vi "high_field_probe_choose_peaks.vi"() -> ()   [LabVIEW 2011]
uses:
  <vilib>/express/express arith-compare/Formula/XNode/ExpressFormulaBlockNode.xnode
  <vilib>/Analysis/NI_AALBase.lvlib
panel:
  out "Zero Ratio":dbl
  out "normalized amplitude":dbl
  out "average power":dbl
  in  "Shutter":bool
  out "Time":string
  in  "3 peak":dbl[](array[numeric])=[0.02, 0.3, 0.12, 0.005, 0.9, 0.012, 0.03, 1.4, 0.12, 0.0]
  in  "3 peaks?":bool
  out "Waveform Chart 2":dbl(graph)
  out "best fit":dbl[](array[numeric])
  in  "Set Zero Peaks":bool
  out "Peak 2 Amp":dbl
  out "Peak 1 Amp":dbl
  out "Polarization":dbl
  out "Peak Ratio":dbl
  out "XY Graph":cluster{dbl[], dbl[]}[](graph)
  in  "Peak 2 at Zero":dbl=1.0
  in  "Peak 1 at Zero":dbl=1.0
  in  "2 peak":dbl[](array[numeric])=[0.02, 0.3, 0.12, 0.03, 1.4, 0.12, 0.0, 1.4, 0.12]
  in  "stop":bool
  in  "Center Freq":dbl=1000.0
  in  "Voltage Sweep Range":dbl=2.2
  out "Set Voltage":dbl
  in  "threshold":dbl=0.0005
  in  "rate":dbl=20000.0
  in  "number of samples":i32=500
  out "data":dynamicdata(graph)
  out "Waveform Chart":dbl(graph)
  out "amplitude":dbl
  out "frequency":dbl
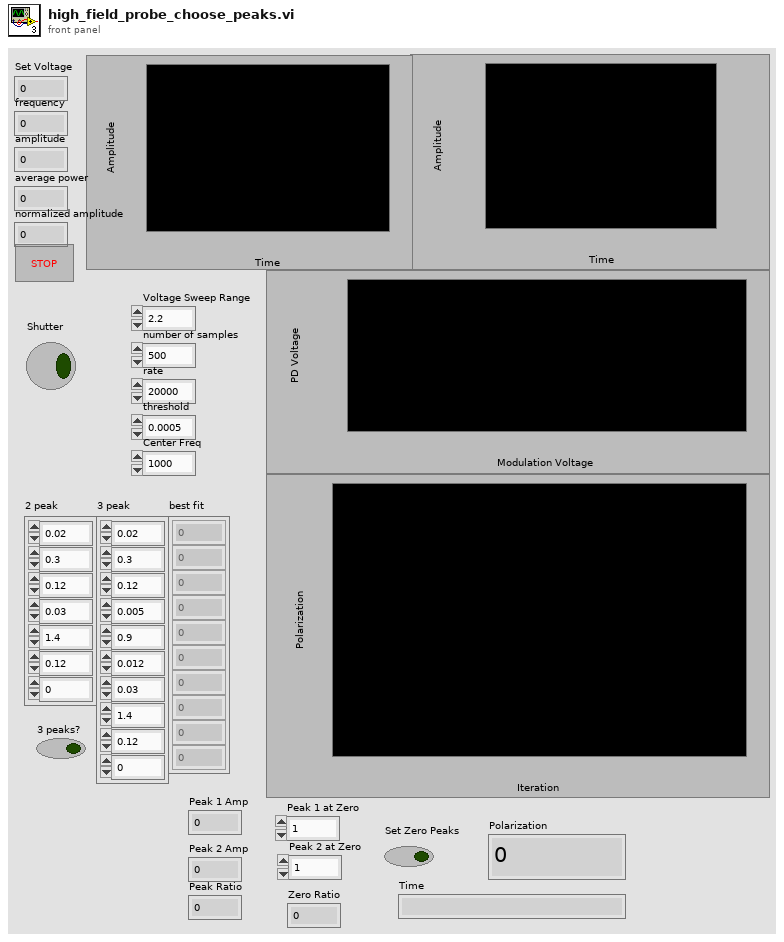
[diagram p1: front panel]
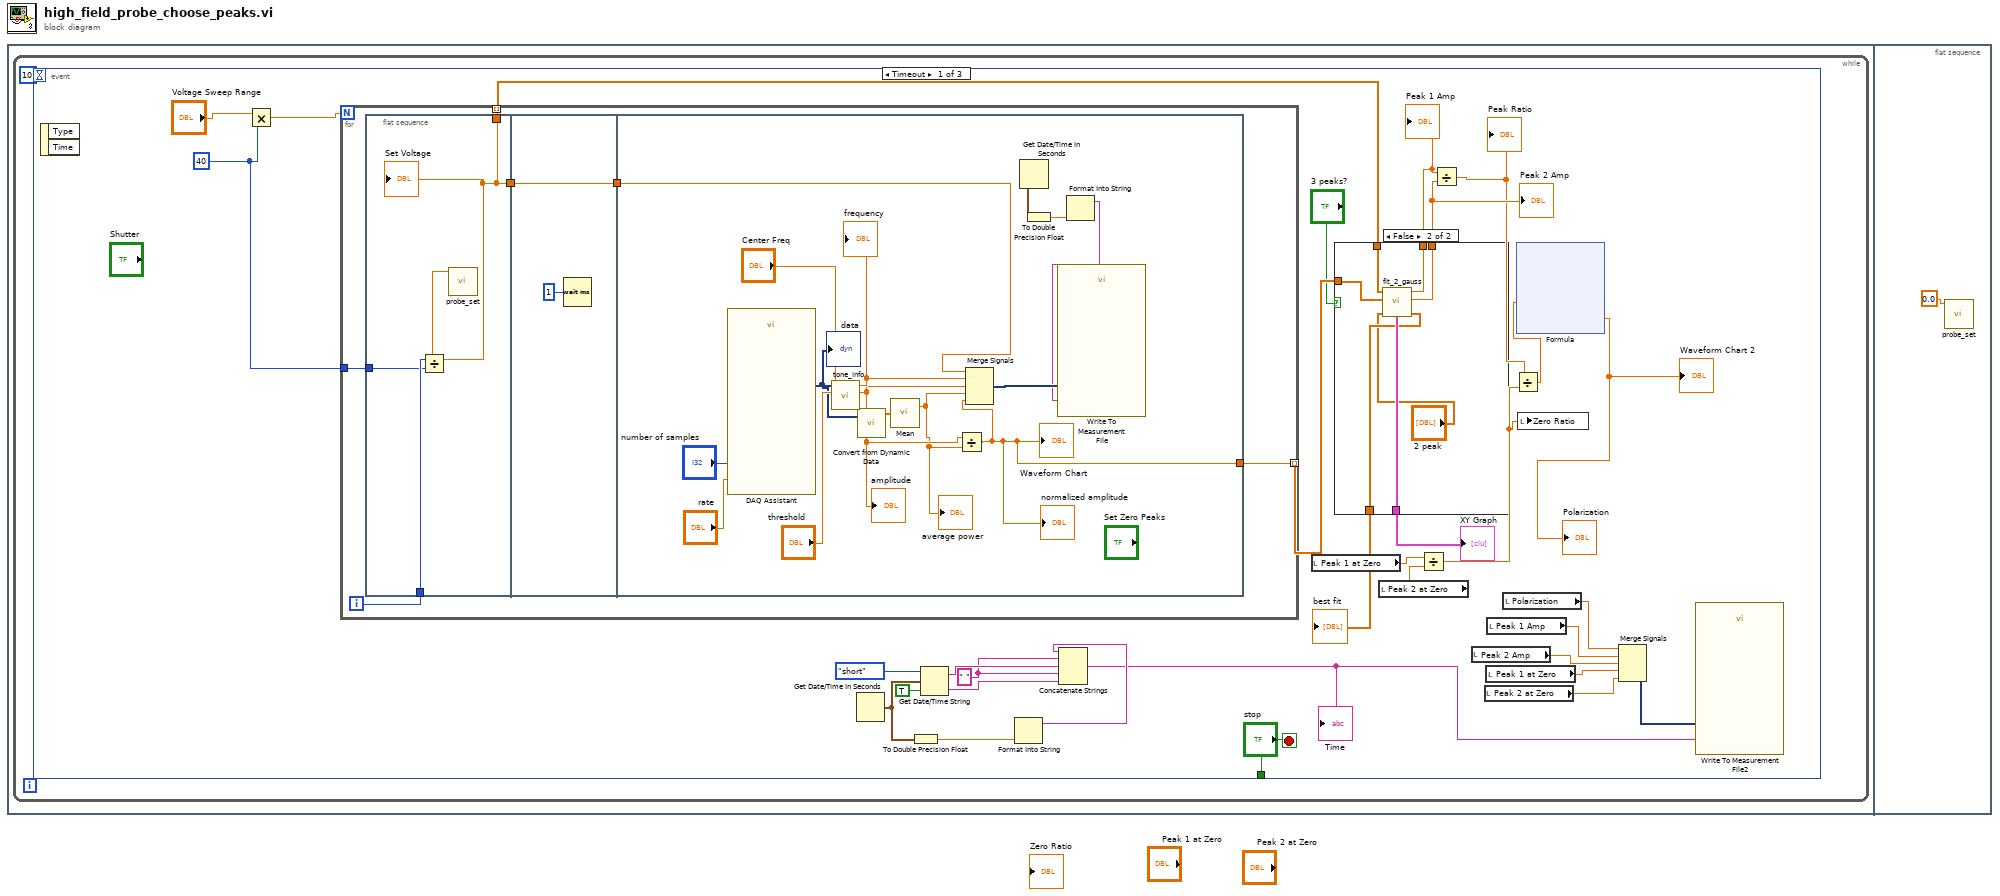
[diagram p0: block diagram]
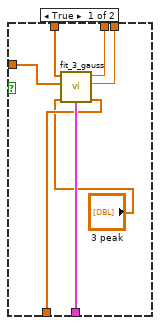
[diagram p2: hidden frame]
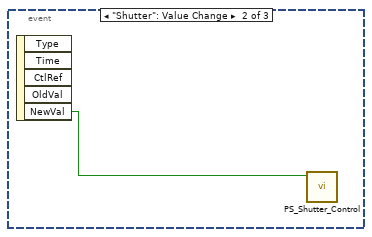
[diagram p3: hidden frame]
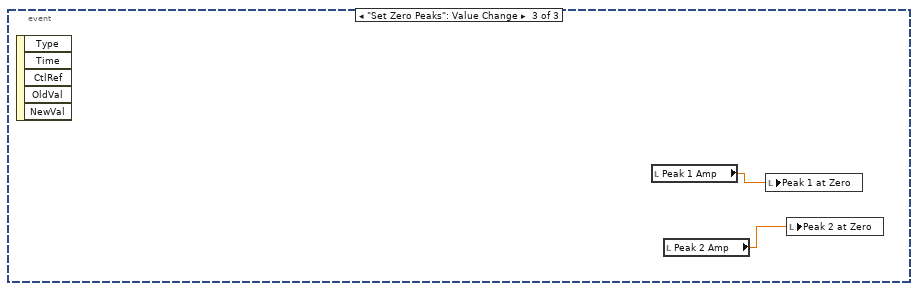
[diagram p4: hidden frame]
diagram:
  n1 = flat-sequence {
    frame #0 {
      n2 = while {
        stop <- w2 stop-if-true
        n3 = event shown="[0] Timeout" {
          selector: _ -> [_ _ _]
          dyn-events: _ -> [_ _ _]
          timeout: 10 -> [_ _ _]
          tunnel: ["stop" _ _] -> w2
          event Timeout {
            w5 = " " ("string")
            w32 = 40 ("y")
            n4 = event-data() -> ()  [unwired: 1 in, 2 out]
            n5 = Multiply(x="Voltage Sweep Range", y=w32) -> (x*y=w33:dbl)
            n6 = for {
              N: w33 -> [_]
              tunnel: w32 -> [w61]
              tunnel: [w58] -> w30 mode=indexing
              tunnel: [w57] -> w29 mode=indexing
              i -> [w62]
              n7 = flat-sequence {
                tunnel: w62 -> [w65]
                tunnel: w61 -> [w64]
                tunnel: [w63] -> w59
                tunnel: [w63] -> w57
                tunnel: [w66] -> w60
                tunnel: w59 -> [w66]
                tunnel: w60 -> [w76]
                tunnel: [w70] -> w58
                frame #0 {
                  n8 = Divide(x=w65, y=w64) -> (x/y=w63:dbl)
                  "Set Voltage" <- w63
                  n9 = call "probe_set.vi"("Voltage"=w63) -> ()  [unwired: 11 in]
                }
                frame #1 {
                  n10 = Wait (ms)(milliseconds to wait=u32 1) -> ()  [unwired: 1 out]
                }
                frame #2 {
                  n11 = call "DAQ Assistant"("rate"="rate", "number of samples"="number of samples") -> ("data"=w72:dynamicdata)  [unwired: 15 in, 2 out]
                  "data" <- w72
                  n12 = call "tone_info.vi"("Center Freq"="Center Freq", "threshold"="threshold", "time signal in"=w72) -> ("amplitude"=w69:dbl, "frequency"=w82:dbl)  [unwired: 6 in, 1 out]
                  "frequency" <- w82
                  "amplitude" <- w69
                  n13 = call "Convert from Dynamic Data"("Dynamic Data Type"=w72) -> ("Array"=w71:dbl[])  [unwired: 3 in]
                  n14 = call <vilib>:"Mean.vi"("X"=w71) -> ("mean"=w68:dbl)  [unwired: 1 out]
                  "average power" <- w68
                  n15 = Divide(x=w69, y=w68) -> (x/y=w70:dbl)
                  "Waveform Chart" <- w70
                  "normalized amplitude" <- w70
                  n16 = Merge Signals(w76, w82, w69, w68, w70) -> (w78:dynamicdata)
                  n17 = Get Date/Time In Seconds() -> (seconds since 1Jan1904=w75:timestamp)
                  n18 = To Double Precision Float(number=w75) -> (double precision float=w74:dbl)
                  n19 = Format Into String(w74) -> (resulting string=w73:string)  [unwired: 3 in, 1 out]
                  n20 = call "Write To Measurement File"("Signals"=w78, "Comment"=w73) -> ()  [unwired: 15 in, 3 out]
                }
              }
            }
            n21 = Get Date/Time In Seconds() -> (seconds since 1Jan1904=w8:timestamp)
            n22 = To Double Precision Float(number=w8) -> (double precision float=w7:dbl)
            n23 = Get Date/Time String(date format (0)=enum16{"short", "long", "abbreviated"}."short", seconds (now)=w8, want seconds? (F)=TRUE) -> (date string=w10:string, time string=w9:string)
            n24 = Format Into String(w7) -> (resulting string=w6:string)  [unwired: 3 in, 1 out]
            n25 = Concatenate Strings(w6, w5, w10, w5, w9) -> (w4:string)
            "Time" <- w4
            n26 = local read "Peak 1 at Zero"() -> (w23:dbl)
            n27 = case shown="False" "3 peaks?" {
              tunnel: w30 -> [w41 w48]
              tunnel: w29 -> [w40 w47]
              tunnel: [w39 w46] -> w28
              tunnel: [w38 w45] -> w27
              tunnel: [w37 w44] -> w26
              tunnel: [w36 w43] -> w20
              frame True {
                n28 = call "fit_3_gauss.vi"("initial parameters"="3 peak", "y Array"=w41, "x Array"=w40) -> ("best fit parameters"=w36:dbl[], "XY Graph"=w37:cluster{dbl[], dbl[]}[], "Peak 3 Amp"=w38:dbl, "Peak 1 Amp"=w39:dbl)  [unwired: 5 in]
              }
              frame False {
                n29 = call "fit_2_gauss.vi"("initial parameters"="2 peak", "y Array"=w48, "x Array"=w47) -> ("best fit parameters"=w43:dbl[], "XY Graph"=w44:cluster{dbl[], dbl[]}[], "Peak 2 Amp"=w45:dbl, "Peak 1 Amp"=w46:dbl)  [unwired: 5 in]
              }
            }
            "XY Graph" <- w26
            "Peak 1 Amp" <- w28
            "Peak 2 Amp" <- w27
            "best fit" <- w20
            n30 = local read "Peak 2 at Zero"() -> (w22:dbl)
            n31 = Divide(x=w23, y=w22) -> (x/y=w3:dbl)
            n32 = Divide(x=w28, y=w27) -> (x/y=w25:dbl)
            "Peak Ratio" <- w25
            n33 = local read "Peak 2 Amp"() -> (w16:dbl)
            n34 = local read "Peak 2 at Zero"() -> (w14:dbl)
            n35 = local read "Peak 1 at Zero"() -> (w15:dbl)
            n36 = local read "Peak 1 Amp"() -> (w17:dbl)
            n37 = local read "Polarization"() -> (w18:dbl)
            n38 = Divide(x=w25, y=w3) -> (x/y=w24:dbl)
            n39 = xnode "Formula"("X"=w24) -> ("Result"=→"Polarization" →"Waveform Chart 2":dbl)  [unwired: 1 in, 1 out]
            n40 = local write "Zero Ratio"(w3) -> ()
            n41 = Merge Signals(w18, w17, w16, w15, w14) -> (w21:dynamicdata)
            n42 = call "Write To Measurement File2"("Signals"=w21, "Comment"=w4) -> ()  [unwired: 15 in, 3 out]
          }
          event "Shutter": Value Change {
            n43 = event-data() -> ("NewVal"=w83:bool)  [unwired: 1 in, 4 out]
            n44 = call "PS_Shutter_Control.vi"("On/Off"=w83) -> ()  [unwired: 10 in, 1 out]
          }
          event "Set Zero Peaks": Value Change {
            n45 = event-data() -> ()  [unwired: 1 in, 5 out]
            n46 = local read "Peak 1 Amp"() -> (w85:dbl)
            n47 = local read "Peak 2 Amp"() -> (w84:dbl)
            n48 = local write "Peak 1 at Zero"(w85) -> ()
            n49 = local write "Peak 2 at Zero"(w84) -> ()
          }
        }
      }
    }
    frame #1 {
      n50 = call "probe_set.vi"("Voltage"=0.0) -> ()  [unwired: 11 in]
    }
  }
